vi "TL Motor MoveAbsolute.vi"() -> ()   [LabVIEW 2012]
doc: "Shows how to move a motor to an absolute position."
panel:
  in  "Abs Pos":dbl
  in  "MG17Motor":refnum<k7>(container)
  in  "Stop":bool
  in  "Set Abs Pos":bool
  in  "MoveAbsolute":bool
  in  "Home":bool
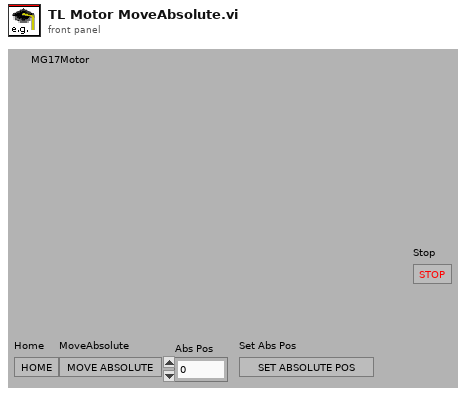
[diagram p1: front panel]
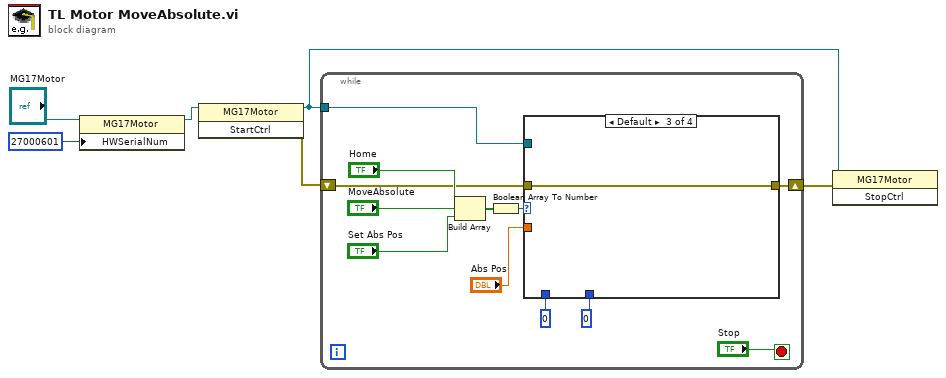
[diagram p0: block diagram]
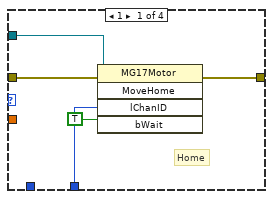
[diagram p2: hidden frame]
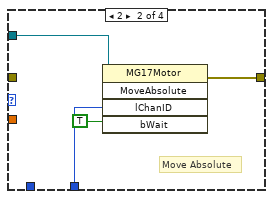
[diagram p3: hidden frame]
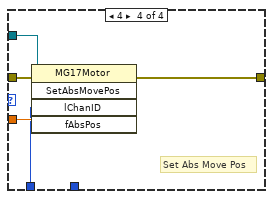
[diagram p4: hidden frame]
diagram:
  n1 = property class="MG17Motor"(reference="MG17Motor", "HWSerialNum"=27000601) -> (reference out=w2:refnum<k7>)  [unwired: 1 in, 1 out]
  n2 = invoke class="MG17Motor" method="StartCtrl"(reference=w2) -> (reference out=w6:refnum<k7>, error out=w5:errorcluster)  [unwired: 2 in, 1 out]
  n3 = while {
    shift-left: w5 -> [w12]
    shift-right: [w13] -> w4
    tunnel: w6 -> [w16]
    stop <- "Stop" stop-if-true
    n4 = Build Array("Home", "MoveAbsolute", "Set Abs Pos") -> (w9:bool[])
    n5 = Boolean Array To Number(Boolean array=w9) -> (number=w10:u32)
    n6 = case shown="Default" w10 {
      tunnel: w16 -> [w23 w27 _ w32]
      tunnel: 0 ("lChanID") -> [w22 w26 _ _]
      tunnel: "Abs Pos" -> [_ _ _ w31]
      tunnel: [w21 w25 w28 w29] -> w13
      tunnel: w12 -> [w20 _ w28 w33]
      tunnel: 0 ("lChanID") -> [_ _ _ w30]
      frame 1 {
        # "Home"
        n7 = invoke class="MG17Motor" method="MoveHome"(reference=w23, error in=w20, "lChanID"=w22, "bWait"=TRUE) -> (error out=w21:errorcluster)  [unwired: 1 in, 4 out]
      }
      frame 2 {
        # "Move Absolute"
        n8 = invoke class="MG17Motor" method="MoveAbsolute"(reference=w27, "lChanID"=w26, "bWait"=TRUE) -> (error out=w25:errorcluster)  [unwired: 2 in, 4 out]
      }
      frame Default {
      }
      frame 4 {
        # "Set Abs Move Pos"
        n9 = invoke class="MG17Motor" method="SetAbsMovePos"(reference=w32, error in=w33, "lChanID"=w30, "fAbsPos"=w31) -> (error out=w29:errorcluster)  [unwired: 1 in, 4 out]
      }
    }
  }
  n10 = invoke class="MG17Motor" method="StopCtrl"(reference=w6, error in=w4) -> ()  [unwired: 1 in, 3 out]
